vi "MoveAnnulusROI.vi"(7 "Action":enum16{"X+", "X-", "Y+", "Y-"}(ring), 8 "error in (no error)":errorcluster, 9 "PItch":i32, 10 "ROI In":T1 {"Contours"."Type" items=["No Selection", "Point", "Line", "Rectangle", "Oval", "Polygon", "Freehand Region", "Annulus", "Unused2", "Unused3", "Broken Line", "Freehand Line", "Rotated Rectangle"]}) -> (0 "error out":errorcluster, 2 "ROI Out":T1 {"Contours"."Type" items=["No Selection", "Point", "Line", "Rectangle", "Oval", "Polygon", "Freehand Region", "Annulus", "Unused2", "Unused3", "Broken Line", "Freehand Line", "Rotated Rectangle"]})   [LabVIEW 2019]
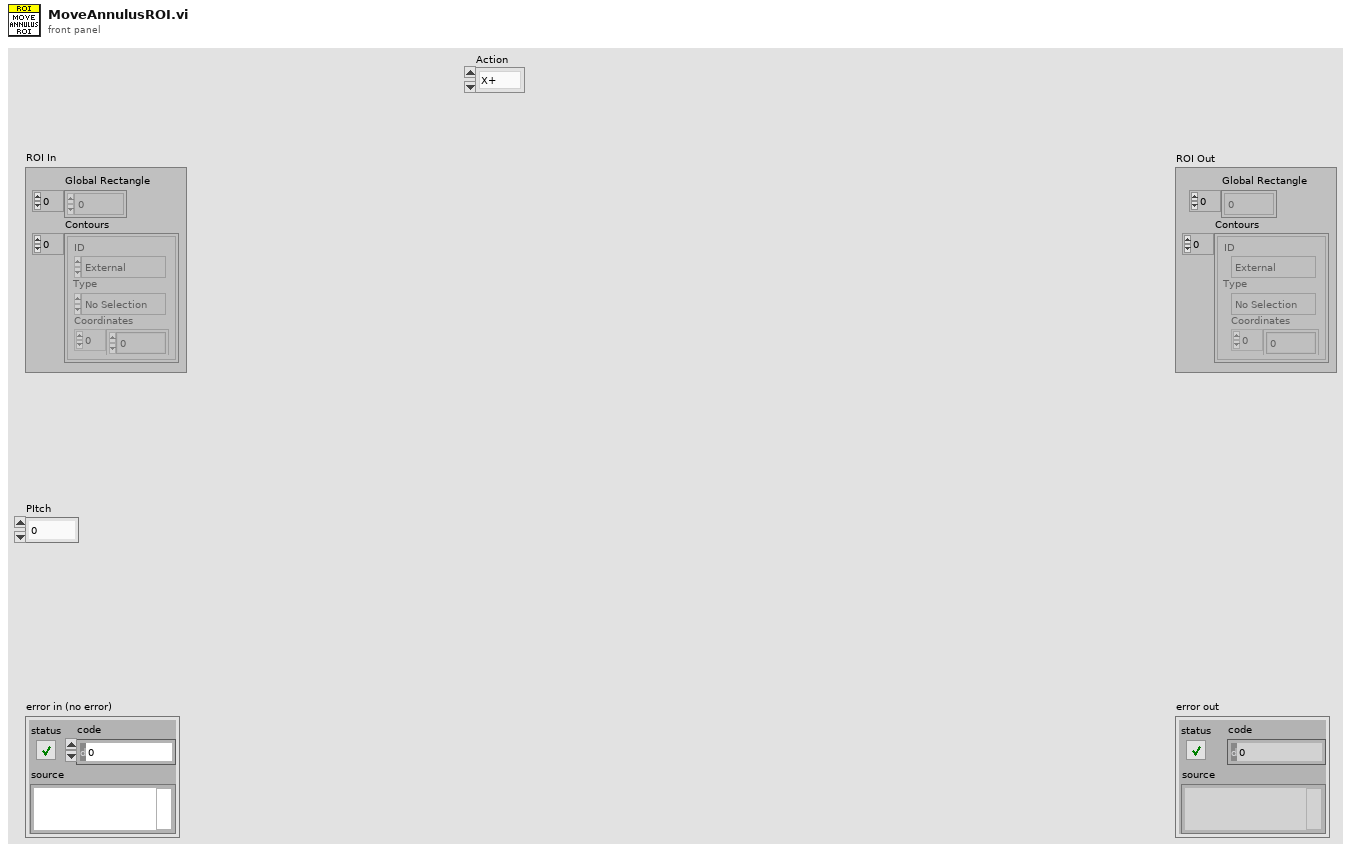
[diagram p1: front panel]
types:
  T1 = typedef "ROI Descriptor" = cluster{"Global Rectangle":i32[], "Contours":cluster{"ID":enum32{"External", "Internal"}, "Type":u32, "Coordinates":i32[]}[]}
  T2 = typedef "IMAQ Circle" = cluster{"Center X":i32, "Center Y":i32, "Inner Radius":i32, "Outer Radius":i32, "Start Angle":dbl, "End Angle":dbl}
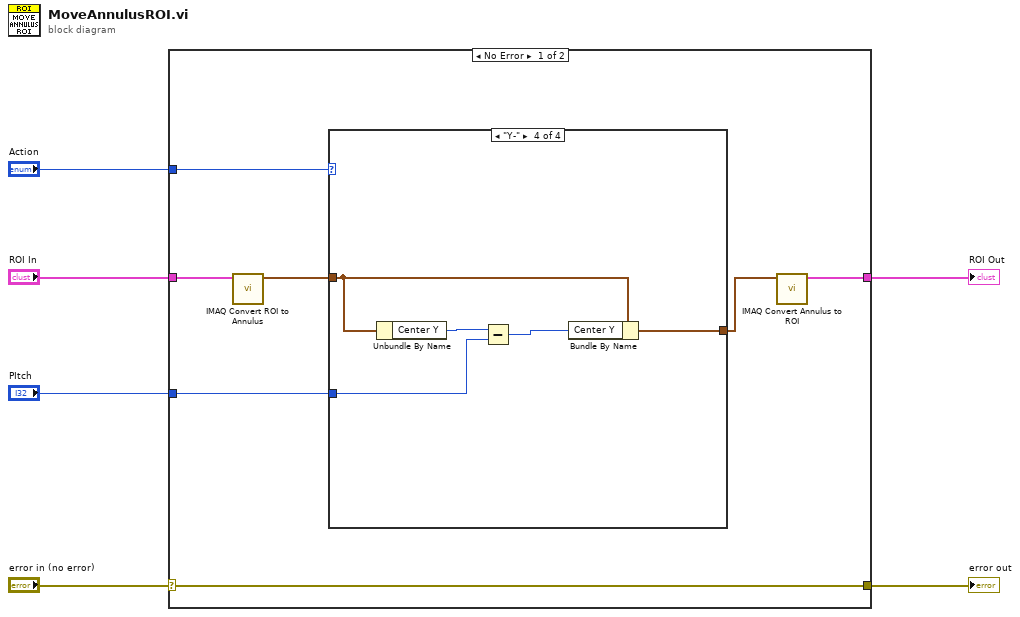
[diagram p0: block diagram]
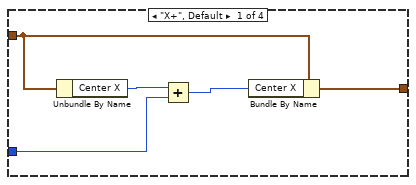
[diagram p2: hidden frame]
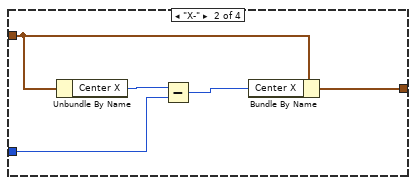
[diagram p3: hidden frame]
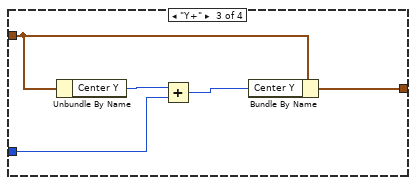
[diagram p4: hidden frame]
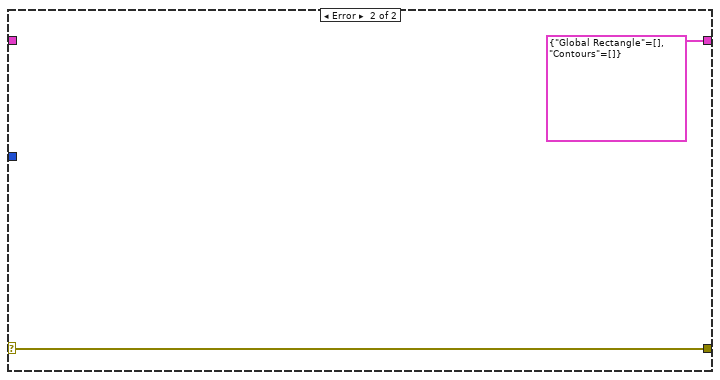
[diagram p5: hidden frame]
diagram:
  n1 = case shown="No Error" "error in (no error)" {
    selector: "error in (no error)" -> [w10 w35]
    tunnel: [w10 w35] -> w5
    tunnel: "Action" -> [w13 _]
    tunnel: "PItch" -> [w12 _]
    tunnel: [w9 T1 {"Global Rectangle"=[], "Contours"=[]} ("ROI Descriptor")] -> w2
    tunnel: "ROI In" -> [w7 _]
    frame No Error {
      n2 = call "IMAQ Convert ROI to Annulus"("ROI Descriptor"=w7) -> ("Annulus"=w8:T2)  [unwired: 8 in, 1 out]
      n3 = case shown="\"Y-\"" w13 {
        tunnel: w8 -> [w15 w23 w25 w33]
        tunnel: w12 -> [w16 w20 w26 w30]
        tunnel: [w14 w19 w24 w29] -> w11
        frame "X+", Default {
          n4 = Unbundle By Name(w15) -> ("Center X"=w18:i32)
          n5 = Add(x=w18, y=w16) -> (x+y=w17:i32)
          n6 = Bundle By Name(cluster=w15, "Center X"=w17) -> (w14:T2)
        }
        frame "X-" {
          n7 = Unbundle By Name(w23) -> ("Center X"=w22:i32)
          n8 = Subtract(x=w22, y=w20) -> (x-y=w21:i32)
          n9 = Bundle By Name(cluster=w23, "Center X"=w21) -> (w19:T2)
        }
        frame "Y+" {
          n10 = Unbundle By Name(w25) -> ("Center Y"=w28:i32)
          n11 = Add(x=w28, y=w26) -> (x+y=w27:i32)
          n12 = Bundle By Name(cluster=w25, "Center Y"=w27) -> (w24:T2)
        }
        frame "Y-" {
          n13 = Unbundle By Name(w33) -> ("Center Y"=w32:i32)
          n14 = Subtract(x=w32, y=w30) -> (x-y=w31:i32)
          n15 = Bundle By Name(cluster=w33, "Center Y"=w31) -> (w29:T2)
        }
      }
      n16 = call "IMAQ Convert Annulus to ROI"("Annulus"=w11) -> ("ROI Descriptor"=w9:T1)  [unwired: 8 in, 1 out]
    }
    frame Error {
    }
  }
  "error out" <- w5
  "ROI Out" <- w2
